vi "test_program_vi.vi"(0 "instrument handle":refnum<k15>, 1 "t_check":dbl, 3 "关断电压":dbl, 4 "中断电压":dbl, 5 "工作频率":dbl caption="Freq", 6 "t_on":dbl, 8 "t_off":dbl, 9 "直流偏置":dbl caption="Dcv", 10 "t_gap":dbl, 11 "工作电压":dbl caption="Acv", 12 "error in (no error)":errorcluster {"code" format="%.0x"}) -> (14 "instrument handle out":refnum<k15>, 15 "error out":errorcluster {"code" format="%.0x"})   [LabVIEW 2020]
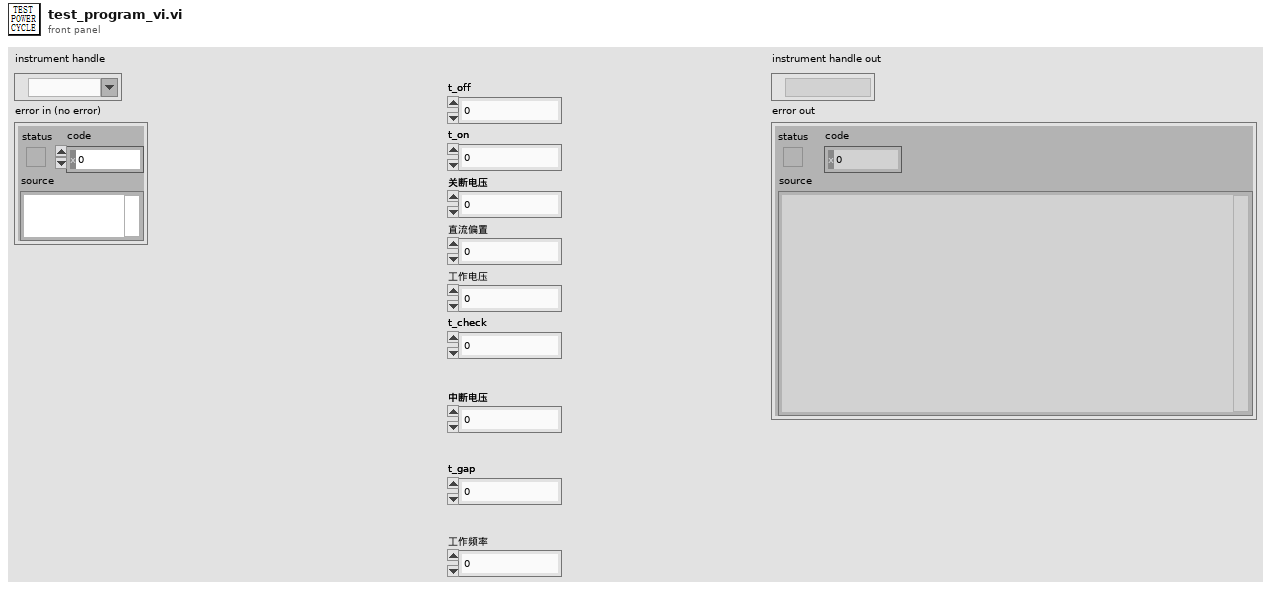
[diagram p1: front panel]
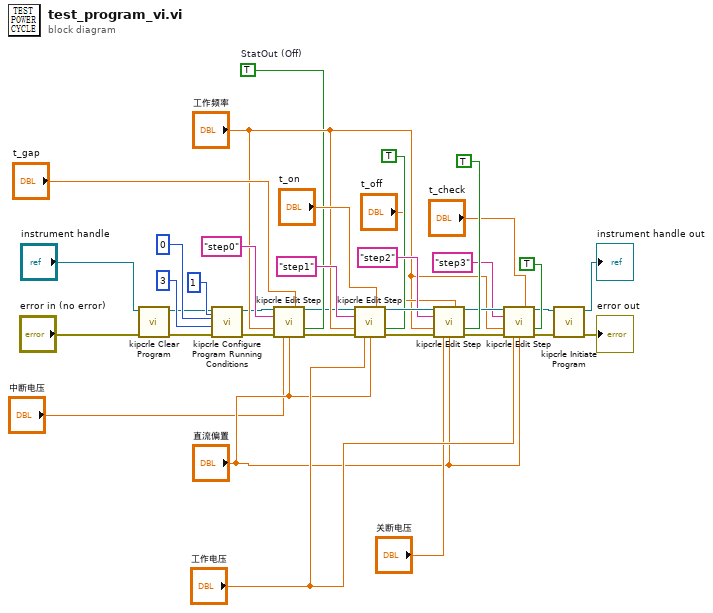
[diagram p0: block diagram]
diagram:
  w7 = TRUE  # StatOut (Off)
  n1 = call <instrlib>:"kipcrle Clear Program.vi"("error in (no error)"="error in (no error)", "instrument handle"="instrument handle") -> ("error out"=w28:errorcluster, "instrument handle out"=w29:refnum<k15>)  [unwired: 8 in]
  n2 = call <instrlib>:"kipcrle Configure Program Running Conditions.vi"("Loop"=1, "error in (no error)"=w28, "EndPosition"=3, "StartPosition"=0, "instrument handle"=w29) -> ("error out"=w3:errorcluster, "instrument handle out"=w6:refnum<k15>)  [unwired: 5 in]
  n3 = call <instrlib>:"kipcrle Edit Step.vi"("instrument handle"=w6, "Time"="t_gap", "Step"="step0", "Freq"="工作频率", "StatOut (Off)"=w7, "error in (no error)"=w3, "Acv"="中断电压", "Dcv"="直流偏置") -> ("instrument handle out"=w5:refnum<k15>, "error out"=w2:errorcluster)  [unwired: 6 in]
  n4 = call <instrlib>:"kipcrle Edit Step.vi"("instrument handle"=w5, "Time"="t_on", "Step"="step1", "Freq"="工作频率", "StatOut (Off)"=TRUE, "error in (no error)"=w2, "Acv"="工作电压", "Dcv"="直流偏置") -> ("instrument handle out"=w26:refnum<k15>, "error out"=w25:errorcluster)  [unwired: 6 in]
  n5 = call <instrlib>:"kipcrle Edit Step.vi"("instrument handle"=w26, "Time"="t_off", "Step"="step2", "Freq"="工作频率", "StatOut (Off)"=TRUE, "error in (no error)"=w25, "Acv"="关断电压", "Dcv"="直流偏置") -> ("instrument handle out"=w21:refnum<k15>, "error out"=w20:errorcluster)  [unwired: 6 in]
  n6 = call <instrlib>:"kipcrle Edit Step.vi"("instrument handle"=w21, "Time"="t_check", "Step"="step3", "Freq"="工作频率", "StatOut (Off)"=TRUE, "error in (no error)"=w20, "Acv"="工作电压", "Dcv"="直流偏置") -> ("instrument handle out"=w4:refnum<k15>, "error out"=w1:errorcluster)  [unwired: 6 in]
  n7 = call <instrlib>:"kipcrle Initiate Program.vi"("error in (no error)"=w1, "instrument handle"=w4) -> ("error out"=→"error out":errorcluster, "instrument handle out"=→"instrument handle out":refnum<k15>)  [unwired: 8 in]
